vi "get_z_intensity tupels.vi"(8 "error in (no error)":errorcluster, 11 "TrajectoryAK101022Resonance in":refnum<class "TrajectoryAK101022Resonance.lvclass">) -> (0 "error out":errorcluster, 1 "z/Intensity tupels OUT":u32[](array[numeric]), 3 "TrajectoryAK101022Resonance out":refnum<class "TrajectoryAK101022Resonance.lvclass">)   [LabVIEW 2010, in "TrajectoryAK101022Resonance.lvclass"]
uses:
  TrajectoryAK101022Resonance.lvclass
  TrajectoryAK101022Resonance.lvclass/TrajectoryAK101022Resonance.ctl
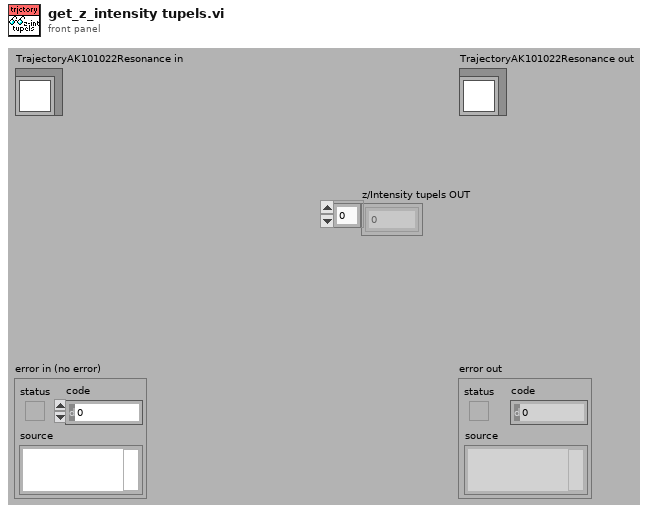
[diagram p1: front panel]
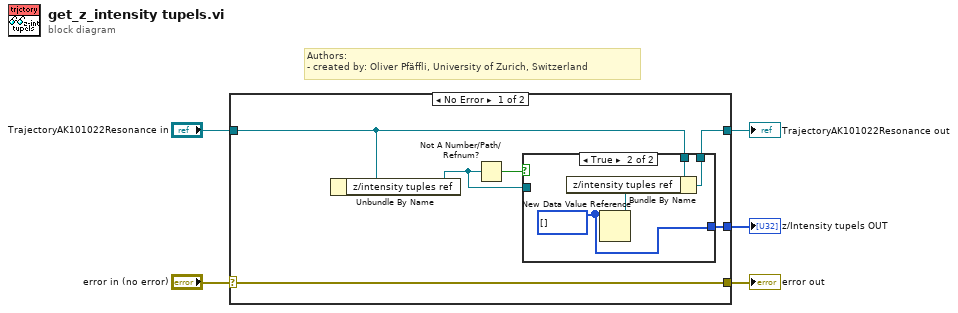
[diagram p0: block diagram]
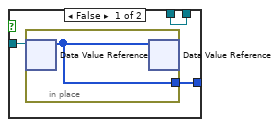
[diagram p2: hidden frame]
diagram:
  # "Authors: \n- created by: Oliver Pfäffli, University of Zurich, Switzerland"
  n1 = case shown="No Error" "error in (no error)" {
    selector: "error in (no error)" -> [w11 w21]
    tunnel: [w11 w21] -> w4
    tunnel: [w8 w20] -> w2
    tunnel: "TrajectoryAK101022Resonance in" -> [w9 w20]
    tunnel: [w6 _] -> w1
    frame No Error {
      n2 = Unbundle By Name(w9) -> ("z/intensity tuples ref"=w7:refnum<data-value>)
      n3 = Not A Number/Path/Refnum?(number/path/refnum=w7) -> (NaN/Path/Refnum?=w10:bool)
      n4 = case shown="True" w10 {
        tunnel: w9 -> [w12 w18]
        tunnel: [w12 w17] -> w8
        tunnel: w7 -> [w14 _]
        tunnel: [w13 w16] -> w6
        frame False {
          n5 = in-place {
            in-place-border: [w15] -> w13
            n6 = in-place-dvr #1(w14) -> (w15:u32[])  [unwired: 1 out]
            n7 = in-place-dvr #1(w15) -> ()  [unwired: 2 out]
          }
        }
        frame True {
          w16 = u32[] []
          n8 = New Data Value Reference(data value=w16) -> (data value reference=w19:refnum<data-value>)  [unwired: 1 in, 1 out]
          n9 = Bundle By Name(cluster=w18, "z/intensity tuples ref"=w19) -> (w17:refnum<class "TrajectoryAK101022Resonance.lvclass">)
        }
      }
    }
    frame Error {
    }
  }
  "error out" <- w4
  "TrajectoryAK101022Resonance out" <- w2
  "z/Intensity tupels OUT" <- w1
